vi "sub_nmea_val.vi"(11 "nmea str":string) -> (2 "checksum":bool, 3 "nmea type":string)   [LabVIEW 2019]
panel:
  out "n":i32
  out "문자열":string
  out "nmea str 3":string
  out "nmea sentence":string
  out "nmea str 2":string
  out "nmea id":string
  out "val":bool
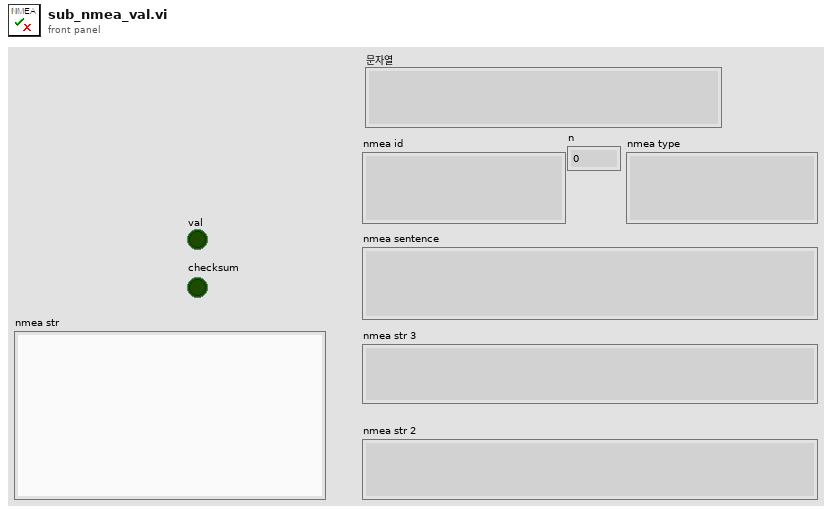
[diagram p1: front panel]
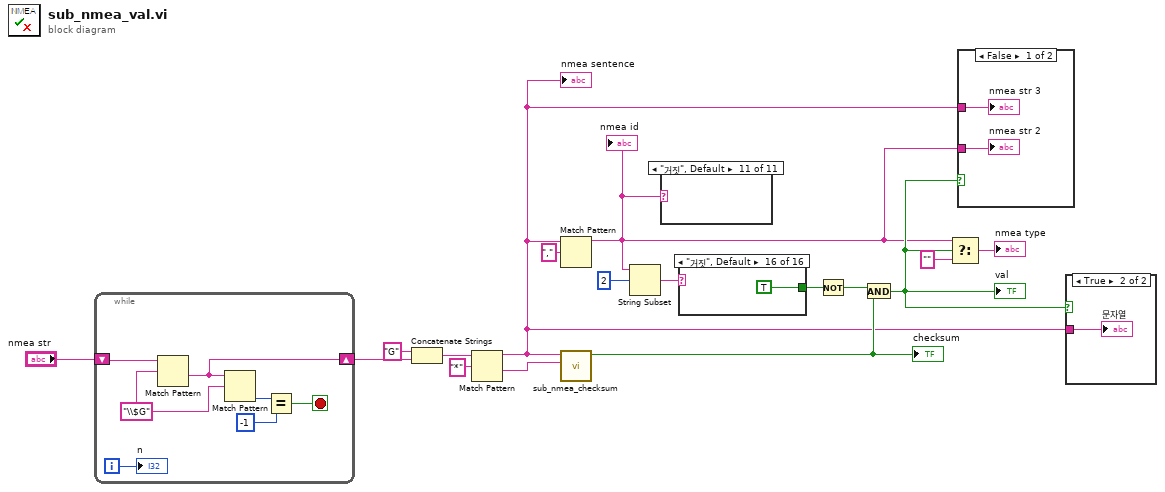
[diagram p0: block diagram]
diagram:
  n1 = while {
    shift-right: [w22] -> w4
    shift-left: "nmea str" -> [w24]
    i -> [w18]
    stop <- w19 stop-if-true
    w23 = "\\$G" ("regular expression")
    n2 = Match Pattern(string=w24, regular expression=w23) -> (after substring=w22:string)  [unwired: 1 in, 3 out]
    n3 = Match Pattern(string=w22, regular expression=w23) -> (offset past match=w21:i32)  [unwired: 1 in, 3 out]
    n4 = Equal?(x=w21, y=-1) -> (x = y?=w19:bool)
    "n" <- w18
  }
  n5 = Concatenate Strings("G" ("문자열"), w4) -> (w6:string)
  n6 = Match Pattern(string=w6, regular expression="*") -> (before substring=w1:string, after substring=w16:string)  [unwired: 1 in, 2 out]
  "nmea sentence" <- w1
  n7 = Match Pattern(string=w1, regular expression="," ("정규식")) -> (before substring=w2:string)  [unwired: 1 in, 3 out]
  "nmea id" <- w2
  n8 = call "sub_nmea_checksum.vi"("nmea checksum"=w16, "nmea raw"=w1) -> ("checksum"=w11:bool)  [unwired: 8 in, 1 out]
  "checksum" <- w11
  n9 = String Subset(string=w2, offset (0)=2 ("오프셋(0)")) -> (substring=w13:string)  [unwired: 1 in]
  n10 = case shown="\"거짓\", Default" w2 {
    frame "GAGSV" {
    }
    frame "GBGSV" {
    }
    frame "GLGSV" {
    }
    frame "GNGGA" {
    }
    frame "GNGLL" {
    }
    frame "GNRMC" {
    }
    frame "GNVTG" {
    }
    frame "GPGGA" {
    }
    frame "GPGSV" {
    }
    frame "GPRMC" {
    }
    frame "거짓", Default {
    }
  }
  n11 = case shown="\"거짓\", Default" w13 {
    tunnel: [_ _ _ _ _ _ _ _ _ _ _ _ _ _ _ TRUE] -> w12
    frame "DTM" {
    }
    frame "GBS" {
    }
    frame "GGA" {
    }
    frame "GLL" {
    }
    frame "GNS" {
    }
    frame "GRS" {
    }
    frame "GSA" {
    }
    frame "GST" {
    }
    frame "GSV" {
    }
    frame "RLM" {
    }
    frame "RMC" {
    }
    frame "THS" {
    }
    frame "TXT" {
    }
    frame "VLW" {
    }
    frame "ZDA" {
    }
    frame "거짓", Default {
    }
  }
  n12 = Not(x=w12) -> (.not. x?=w10:bool)
  n13 = And(x=w10, y=w11) -> (x .and. y?=w3:bool)
  "val" <- w3
  n14 = Select(t=w2, s=w3, f="") -> (s? t:f=→"nmea type":string)
  n15 = case shown="False" w3 {
    tunnel: w2 -> [w27 _]
    tunnel: w1 -> [w26 _]
    frame False {
      "nmea str 2" <- w27
      "nmea str 3" <- w26
    }
    frame True {
    }
  }
  n16 = case shown="True" w3 {
    tunnel: w1 -> [_ w28]
    frame False {
    }
    frame True {
      "문자열" <- w28
    }
  }
